vi "Class Arr to Tree Arr.vi"(11 "Sorted Classes":T1(array[cluster])) -> (3 "Array":T2[](array[typedef]))   [LabVIEW 2023]
uses:
  Class Item Cluster.ctl
  controls/action enum.ctl
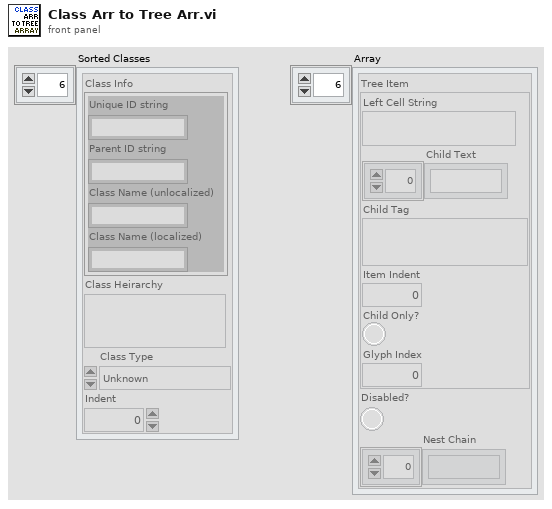
[diagram p1: front panel]
types:
  T1 = cluster{"Class Info":cluster{"Unique ID string":string, "Parent ID string":string, "Class Name (unlocalized)":string, "Class Name (localized)":string}, "Class Heirarchy":string, "Class Type":enum16{"Unknown", "Base", "Scripting", "Private", "Deprecated", "None", "Divider"}, "Indent":u32}[]
  T2 = typedef "Class Item Cluster.ctl" = cluster{"Tree Item":cluster{"Left Cell String":string, "Child Text":string[], "Child Tag":string, "Item Indent":i32, "Child Only?":bool, "Glyph Index":i32}, "Disabled?":bool, "Nest Chain":string[]}
  T3 = typedef "action enum.ctl" = enum16{"[NONE]", "APP_SEPARATOR", "Wire Bundle", "Wire Unbundle", "Terminal Unbundle", "Terminal Bundle", "Bundler Move Up", "Bundler Move Down", "Bundler Insert", "Bundler Remove", "Bundler Remove Unwired", "Bundler Reorder", "In Place Insert", "In Place Remove", "In Place Remove Unwired", "In Place Reorder", "Wire Properties", "Wire Method", "Terminal Properties", "Terminal Method", "Property Move Up", "Property Move Down", "Properties Insert", "Properties Remove", "Properties Remove Unwired", "Properties Reorder", "Method Change", "Class For Constant", "Class For Control", "Class For Node", "Class Name to Clipboard"}
  T4 = enum16{"Unknown", "Base", "Scripting", "Private", "Deprecated", "None", "Divider"}
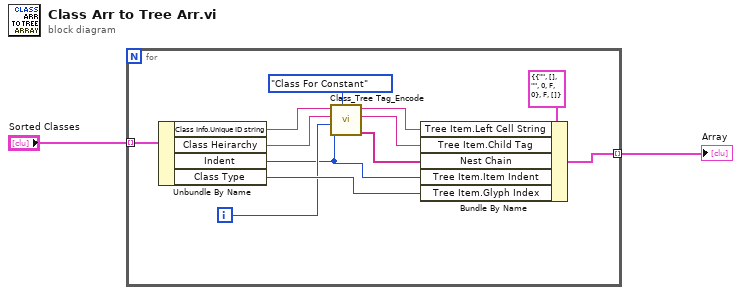
[diagram p0: block diagram]
diagram:
  n1 = for {
    tunnel: "Sorted Classes" -> [w13] mode=indexing
    tunnel: [w14] -> w2 mode=indexing
    i -> [w8]
    n2 = Unbundle By Name(w13) -> ("Class Info.Unique ID string"=w10:string, "Class Heirarchy"=w9:string, "Indent"=w7:u32, "Class Type"=w12:T4)
    n3 = call "Class_Tree Tag_Encode.vi"("Action"=action_enum."Class For Constant", "Property Type"=w7, "Index"=w8, "Hierarchy"=w9, "Unique ID string"=w10) -> ("Parents"=w4:string[], "Tag"=w5:string, "Display name"=w6:string)  [unwired: 3 in, 1 out]
    n4 = Bundle By Name(cluster=T2 {"Tree Item"={"Left Cell String"="", "Child Text"=[], "Child Tag"="", "Item Indent"=0, "Child Only?"=FALSE, "Glyph Index"=0}, "Disabled?"=FALSE, "Nest Chain"=[]} ("Property For Tree with Disabled"), "Tree Item.Left Cell String"=w6, "Tree Item.Child Tag"=w5, "Nest Chain"=w4, "Tree Item.Item Indent"=w7, "Tree Item.Glyph Index"=w12) -> (w14:T2)
  }
  "Array" <- w2
